vi "TurnOffRobcommACI.vi"(2 "error in":errorcluster, 4 "VISA resource name":refnum<visa-resource-name>="COM1") -> (0 "error out 2":errorcluster)   [LabVIEW 2012]
uses:
  <vilib>/Instr/_visa.llb/VISA Open Access Mode.ctl
  <vilib>/Instr/_visa.llb/VISA Configure Serial Port (Instr).vi
panel:
  out "READ ACK":string
  out "read buffer 2":string
  out "read buffer":string
  out "STATUS OUT":u32
  out "eighth bytes out":u32
  out "status out":string
  out "seventh bytes out":u32
  out "sixth bytes out":u32
  out "fifth bytes out":u32
  out "fourth bytes out":u32
  out "third bytes out":u32
  out "second bytes out":u32
  out "first bytes out":u32
  in  "close com1":bool=TRUE
  out "FIRST READ":string
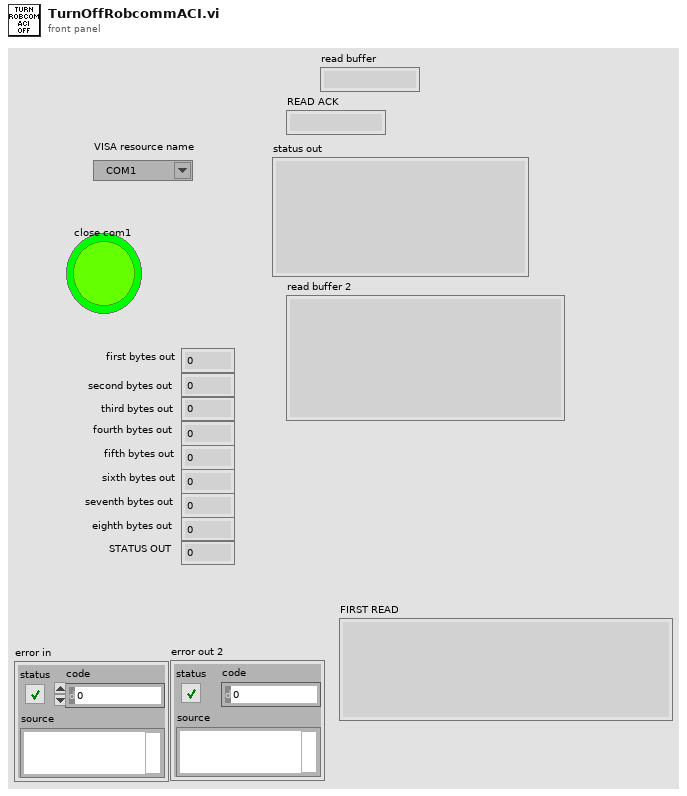
[diagram p1: front panel]
types:
  T1 = typedef "VISA Open Access Mode.ctl" = u32
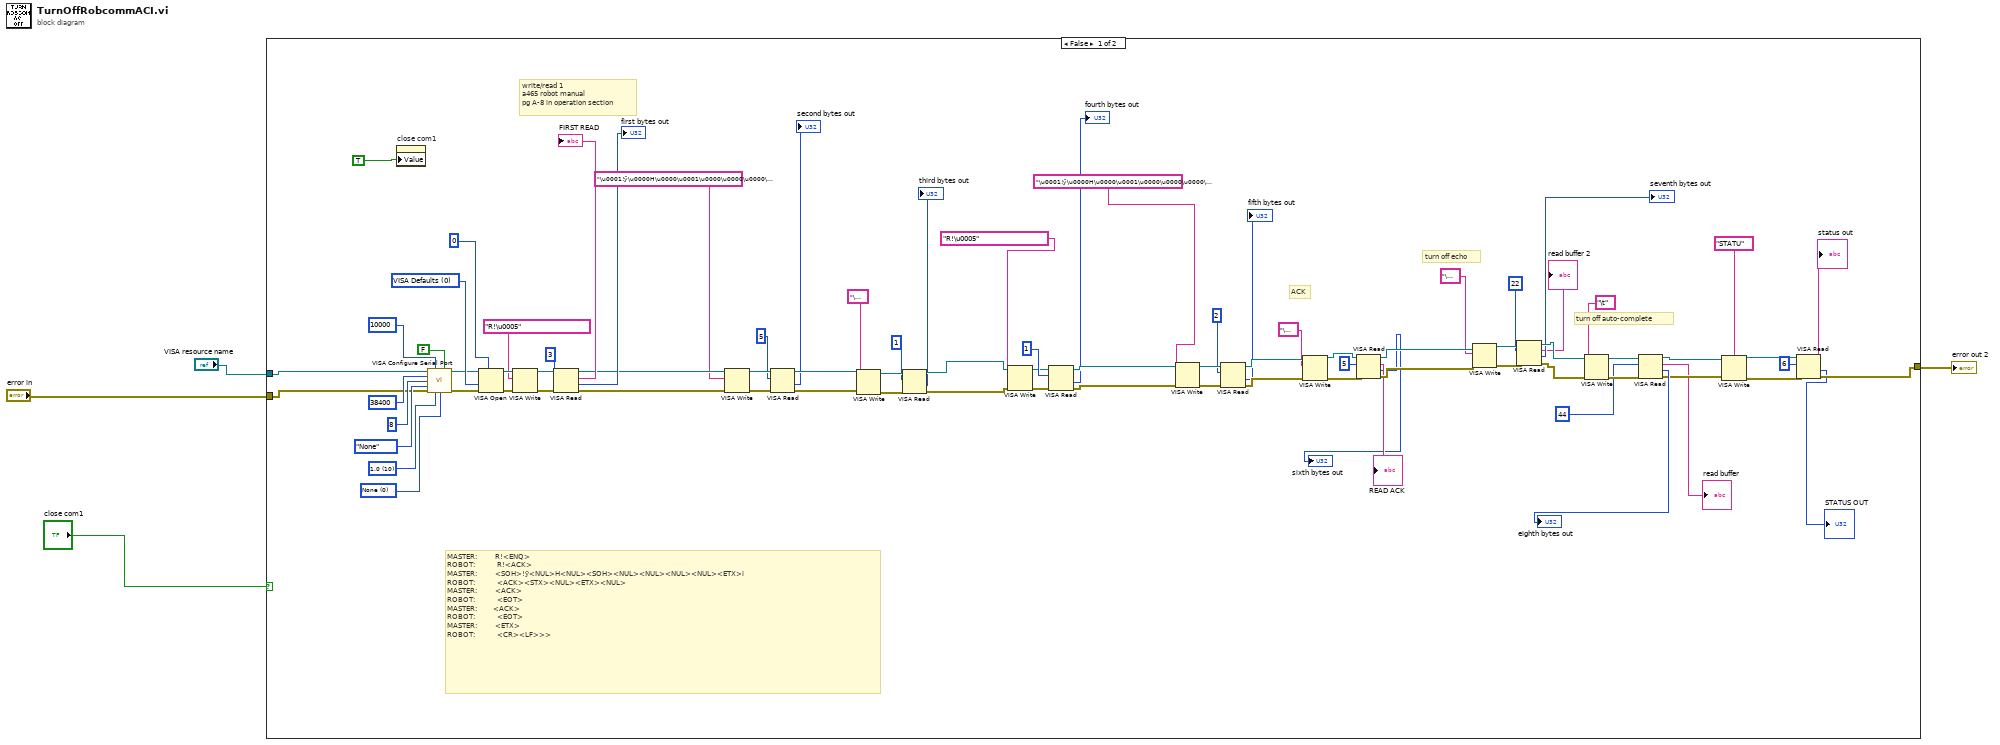
[diagram p0: block diagram]
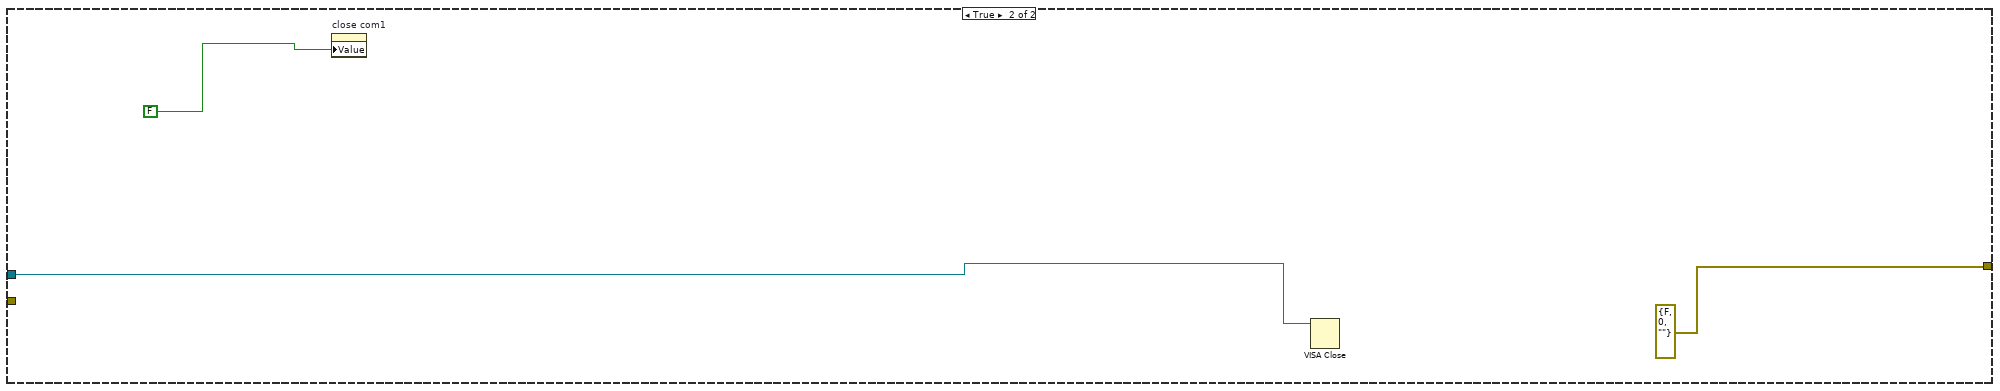
[diagram p2: hidden frame]
diagram:
  n1 = case shown="False" "close com1" {
    tunnel: "VISA resource name" -> [w35 w89]
    tunnel: [w28 errorcluster {"status"=FALSE, "code"=0, "source"=""} ("error out")] -> w2
    tunnel: "error in" -> [w12 _]
    frame False {
      w77 = u16 0 items=["None", "XON/XOFF", "RTS/CTS", "XON/XOFF & RTS/CTS", "DTR/DSR", "XON/XOFF & DTR/DSR"] ("flow control (0:none)")
      w78 = u16 10 items=["1.0"=10, "1.5"=15, "2.0"=20] ("stop bits (10: 1 bit)")
      w83 = T1 0 items=["VISA Defaults"=0, "Exclusive Lock"=1, "Load Configured Settings"=4] ("Access Mode")
      # "ACK"
      # "turn off auto-complete"
      # "turn off echo"
      # "MASTER:         R!<ENQ>\nROBOT:           R!<ACK>\nMASTER:         <SOH>!ÿ<NUL>H<NUL><SOH><NUL><NUL><NUL><NUL><ETX>i\nROBOT:           <ACK><STX><NUL><ETX><NUL>\nMASTER:         <ACK>\nROBOT:           <EOT>\nMASTER:        <ACK>\nROBOT:           <EOT>\nMASTER:         <ETX>\nROBOT:           <CR><LF>>>"
      # "write/read 1\na465 robot manual\npg A-8 in operation section"
      n2 = property on="close com1" class="Bool (strict)"("Value"=TRUE) -> ()  [unwired: 2 in, 2 out]
      n3 = call-poly "VISA Configure Serial Port"("VISA resource name"=w35, "timeout (10sec)"=u32 10000, "Enable Termination\nChar (T)"=FALSE ("Enable Termination\nChar (T)"), "baud rate (9600)"=u32 38400, "data bits (8)"=u16 8, "parity (0:none)"=enum16{"None", "Odd", "Even", "Mark", "Space"}."None", "error in (no error)"=w12, "stop bits (10: 1 bit)"=w78, "flow control (0:none)"=w77) -> ("VISA resource name out"=w79:refnum<visa-resource-name>, "error out"=w74:errorcluster)  [unwired: 5 in]
      n4 = VISA Open(timeout (0)=u32 0 ("VISA Open timeout (0)"), access mode=w83, error in (no error)=w74, VISA resource name=w79) -> (VISA resource name=w84:refnum<visa-resource-name>, error out=w73:errorcluster)  [unwired: 1 in]
      n5 = VISA Write(VISA resource name=w84, write buffer="R!\u0005", error in (no error)=w73) -> (VISA resource name out=w87:refnum<visa-resource-name>, error out=w85:errorcluster)  [unwired: 1 out]
      n6 = VISA Read(VISA resource name=w87, byte count=u32 3, error in (no error)=w85) -> (VISA resource name out=w70:refnum<visa-resource-name>, read buffer=→"FIRST READ":string, return count=→"first bytes out":u32, error out=w43:errorcluster)
      n7 = VISA Write(VISA resource name=w70, write buffer="\u0001!ÿ\u0000H\u0000\u0001\u0000\u0000\u0000\u0000\u0003i" ("write buffer 2"), error in (no error)=w43) -> (VISA resource name out=w66:refnum<visa-resource-name>, error out=w67:errorcluster)  [unwired: 1 out]
      n8 = VISA Read(VISA resource name=w66, byte count=u32 5, error in (no error)=w67) -> (VISA resource name out=w64:refnum<visa-resource-name>, return count=→"second bytes out":u32, error out=w63:errorcluster)  [unwired: 1 out]
      n9 = VISA Write(VISA resource name=w64, write buffer="\u0006", error in (no error)=w63) -> (VISA resource name out=w62:refnum<visa-resource-name>, error out=w61:errorcluster)  [unwired: 1 out]
      n10 = VISA Read(VISA resource name=w62, byte count=u32 1, error in (no error)=w61) -> (VISA resource name out=w57:refnum<visa-resource-name>, return count=→"third bytes out":u32, error out=w55:errorcluster)  [unwired: 1 out]
      n11 = VISA Write(VISA resource name=w57, write buffer="R!\u0005", error in (no error)=w55) -> (VISA resource name out=w58:refnum<visa-resource-name>, error out=w54:errorcluster)  [unwired: 1 out]
      n12 = VISA Read(VISA resource name=w58, byte count=u32 1, error in (no error)=w54) -> (VISA resource name out=w53:refnum<visa-resource-name>, return count=→"fourth bytes out":u32, error out=w52:errorcluster)  [unwired: 1 out]
      n13 = VISA Write(VISA resource name=w53, write buffer="\u0001!ÿ\u0000H\u0000\u0001\u0000\u0000\u0000\u0000\u0003i" ("write buffer 2"), error in (no error)=w52) -> (VISA resource name out=w50:refnum<visa-resource-name>, error out=w51:errorcluster)  [unwired: 1 out]
      n14 = VISA Read(VISA resource name=w50, byte count=u32 2, error in (no error)=w51) -> (VISA resource name out=w48:refnum<visa-resource-name>, return count=→"fifth bytes out":u32, error out=w47:errorcluster)  [unwired: 1 out]
      n15 = VISA Write(VISA resource name=w48, write buffer="\u0006", error in (no error)=w47) -> (VISA resource name out=w8:refnum<visa-resource-name>, error out=w10:errorcluster)  [unwired: 1 out]
      n16 = VISA Read(VISA resource name=w8, byte count=u32 5, error in (no error)=w10) -> (VISA resource name out=w46:refnum<visa-resource-name>, read buffer=→"READ ACK":string, return count=→"sixth bytes out":u32, error out=w45:errorcluster)
      n17 = VISA Write(VISA resource name=w46, write buffer="\u0005", error in (no error)=w45) -> (VISA resource name out=w26:refnum<visa-resource-name>, error out=w25:errorcluster)  [unwired: 1 out]
      n18 = VISA Read(VISA resource name=w26, byte count=u32 22, error in (no error)=w25) -> (VISA resource name out=w23:refnum<visa-resource-name>, read buffer=→"read buffer 2":string, return count=→"seventh bytes out":u32, error out=w24:errorcluster)
      n19 = VISA Write(VISA resource name=w23, write buffer="\t", error in (no error)=w24) -> (VISA resource name out=w18:refnum<visa-resource-name>, error out=w19:errorcluster)  [unwired: 1 out]
      n20 = VISA Read(VISA resource name=w18, byte count=u32 44, error in (no error)=w19) -> (VISA resource name out=w17:refnum<visa-resource-name>, read buffer=→"read buffer":string, return count=→"eighth bytes out":u32, error out=w15:errorcluster)
      n21 = VISA Write(VISA resource name=w17, write buffer="STATU", error in (no error)=w15) -> (VISA resource name out=w33:refnum<visa-resource-name>, error out=w34:errorcluster)  [unwired: 1 out]
      n22 = VISA Read(VISA resource name=w33, byte count=u32 6, error in (no error)=w34) -> (read buffer=→"status out":string, return count=→"STATUS OUT":u32, error out=w28:errorcluster)  [unwired: 1 out]
    }
    frame True {
      n23 = property on="close com1" class="Bool (strict)"("Value"=FALSE) -> ()  [unwired: 2 in, 2 out]
      n24 = VISA Close(VISA resource name=w89) -> ()  [unwired: 1 in, 1 out]
    }
  }
  "error out 2" <- w2
